vi "Hardware-RegisterFaultPoints.vi"(8 "System State":T3 {"System ADC"."Fan [V]" format="%#_3p"; "System ADC"."Primary B1B2 [V]" format="%#_3p"; "System ADC"."Primary B3B4 [V]" format="%#_3p"; "System ADC"."Primary A3A4 [V]" format="%#_3p"; "System ADC"."Primary A1A2 [V]" format="%#_3p"; "System ADC"."MPRD [V]" format="%#_3p"; "System ADC"."Ext HV B [V]" format="%#_3p"; "System ADC"."Ext HV A [V]" format="%#_3p"; "System ADC"."Pump Zener B [V]" format="%#_3p"; "System ADC"."Pump Zener A [V]" format="%#_3p"; "System ADC"."DI Zener B [V]" format="%#_3p"; "System ADC"."DI Zener A [V]" format="%#_3p"; "System ADC"."Key [V]" format="%#_3p"; "System ADC"."DRVP [V]" format="%#_3p"; "System ADC"."Battery [V]" format="%#_3p"; "System ADC"."FET Driver [V]" format="%#_3p"; "System ADC"."Secondary B1B2 [V]" format="%#_3p"; "System ADC"."Secondary B3B4 [V]" format="%#_3p"; "System ADC"."Secondary A3A4 [V]" format="%#_3p"; "System ADC"."Secondary A1A2 [V]" format="%#_3p"; "System ADC"."Primary Range [V]" format="%#_3p"; "System ADC"."Temp Boost B [C]" format="%#_3p"; "System ADC"."Temp Primary A [C]" format="%#_3p"; "System ADC"."Temp Secondary A [C]" format="%#_3p"; "System ADC"."Temp Fan Intake [C]" format="%#_3p"; "System ADC"."Temp CPU [C]" format="%#_3p"; "System ADC"."Temp DI Zener B [C]" format="%#_3p"; "System ADC"."Temp DI B [C]" format="%#_3p"; "System ADC"."Temp DI Zener A [C]" format="%#_3p"; "System ADC"."Temp DI A [C]" format="%#_3p"; "System ADC"."Temp HH 7-12 [C]" format="%#_3p"; "System ADC"."Temp HH 1-6 [C]" format="%#_3p"; "System ADC"."AI 12 [V]" format="%#_3p"; "System ADC"."AI 11 [V]" format="%#_3p"; "System ADC"."AI 10 [V]" format="%#_3p"; "System ADC"."AI 9 [V]" format="%#_3p"; "System ADC"."AI 8 [V]" format="%#_3p"; "System ADC"."AI 7 [V]" format="%#_3p"; "System ADC"."AI 6 [V]" format="%#_3p"; "System ADC"."AI 5 [V]" format="%#_3p"; "System ADC"."AI 4 [V]" format="%#_3p"; "System ADC"."AI 3 [V]" format="%#_3p"; "System ADC"."AI 2 [V]" format="%#_3p"; "System ADC"."AI 1 [V]" format="%#_3p"}, 9 "DI-B Faults":T1, 10 "DI-A Faults":T1, 11 "HH Status":T6[](array[typedef]) {"On Avg [A]" format="%#_6p"; "Period Avg [A]" format="%#_6p"; "Period Max [A]" format="%#_6p"; "Period Min [A]" format="%#_6p"}) -> ()   [LabVIEW 2016, in "DSI-RT.lvlib"]
uses:
  DSI-RT.lvlib
  <vilib>/Powertrain Controls/Device Drivers/DCM/HH/RT/Status.ctl
  <vilib>/Powertrain Controls/Device Drivers/DCM/Rev0/RT/System State.ctl
  <vilib>/Powertrain Controls/Device Drivers/DCM/Rev0/RT/System ADC.ctl
  <vilib>/Powertrain Controls/Device Drivers/DCM/Rev0/RT/Internal Fault.ctl
  Shared/Typedefs/DI-Faults-Array.ctl
  <vilib>/Powertrain Controls/Device Drivers/DCM/Rev0/FPGA/DI - Faults.ctl
  <vilib>/addons/Software Calibration Management/xSCM/FaultPoint.xnode
  <vilib>/addons/Software Calibration Management/xSCM/CalPoint.xnode
  <vilib>/addons/Software Calibration Management/xSCM/ni_scm.dll
  <vilib>/Powertrain Controls/Device Drivers/DCM/Rev0/RT/DCM - RT.lvclass
  <vilib>/Powertrain Controls/Device Drivers/DCM/HH/RT/DCM - RT - HH.lvlib
  <vilib>/Powertrain Controls/Device Drivers/DCM/Rev0/FPGA/DCM - FPGA.lvlib
  Shared/DSI-Shared.lvlib
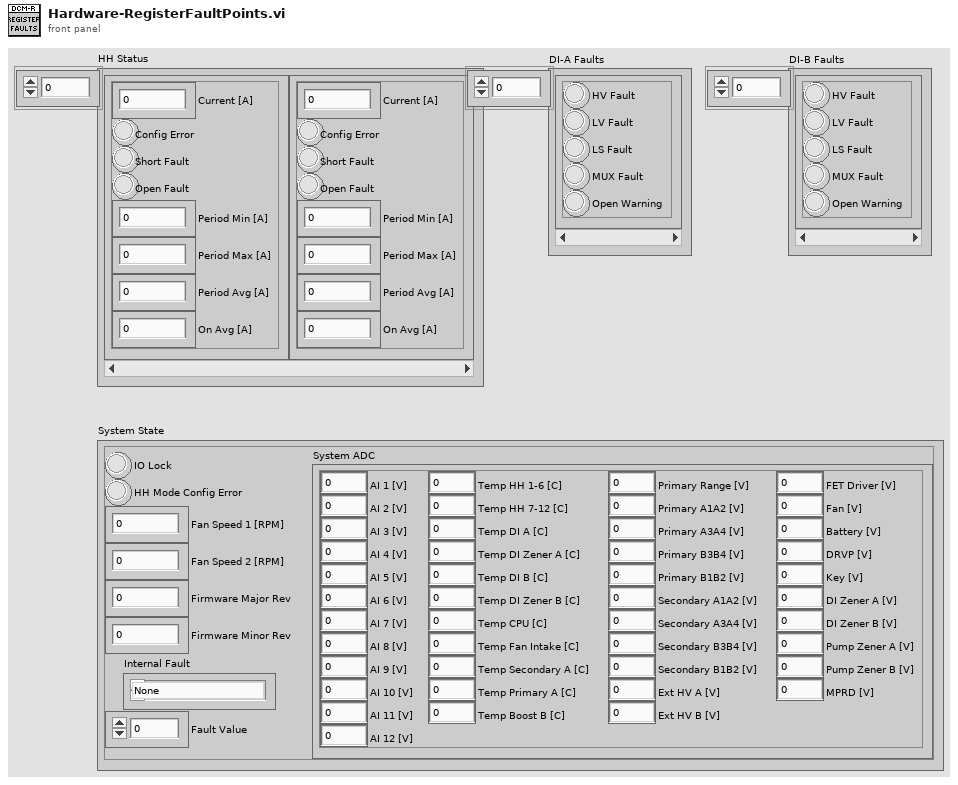
[diagram p1: front panel]
types:
  T1 = typedef "DSI-Shared.lvlib/DI-Faults-Array.ctl" = T2[]
  T2 = typedef "DCM - FPGA.lvlib/DI - Faults.ctl" = cluster{"HV Fault":bool, "LV Fault":bool, "LS Fault":bool, "MUX Fault":bool, "Open Warning":bool}
  T3 = typedef "DCM - RT.lvclass/System State.ctl" = cluster{"System ADC":T4, "IO Lock":bool, "HH Mode Config Error":bool, "Fan Speed 1 [RPM]":sgl, "Fan Speed 2 [RPM]":sgl, "Firmware Major Rev":u16, "Firmware Minor Rev":u16, "Internal Fault":T5, "Fault Value":dbl}
  T4 = typedef "DCM - RT.lvclass/System ADC.ctl" = cluster{"AI 1 [V]":sgl, "AI 2 [V]":sgl, "AI 3 [V]":sgl, "AI 4 [V]":sgl, "AI 5 [V]":sgl, "AI 6 [V]":sgl, "AI 7 [V]":sgl, "AI 8 [V]":sgl, "AI 9 [V]":sgl, "AI 10 [V]":sgl, "AI 11 [V]":sgl, "AI 12 [V]":sgl, "Temp HH 1-6 [C]":sgl, "Temp HH 7-12 [C]":sgl, "Temp DI A [C]":sgl, "Temp DI Zener A [C]":sgl, "Temp DI B [C]":sgl, "Temp DI Zener B [C]":sgl, "Temp CPU [C]":sgl, "Temp Fan Intake [C]":sgl, "Temp Secondary A [C]":sgl, "Temp Primary A [C]":sgl, "Temp Boost B [C]":sgl, "Primary Range [V]":sgl, "Primary A1A2 [V]":sgl, "Primary A3A4 [V]":sgl, "Primary B3B4 [V]":sgl, "Primary B1B2 [V]":sgl, "Secondary A1A2 [V]":sgl, "Secondary A3A4 [V]":sgl, "Secondary B3B4 [V]":sgl, "Secondary B1B2 [V]":sgl, "Ext HV A [V]":sgl, "Ext HV B [V]":sgl, "FET Driver [V]":sgl, "Fan [V]":sgl, "Battery [V]":sgl, "DRVP [V]":sgl, "Key [V]":sgl, "DI Zener A [V]":sgl, "DI Zener B [V]":sgl, "Pump Zener A [V]":sgl, "Pump Zener B [V]":sgl, "MPRD [V]":sgl}
  T5 = typedef "DCM - RT.lvclass/Internal Fault.ctl" = enum32{"None", "Temp HH 1-6", "Temp HH 7-12", "Temp DI A", "Temp DI Zener A", "Temp DI B", "Temp DI Zener B", "Temp Intake", "Temp Primary A", "Temp Secondary A", "Temp Boost B", "Temp CPU", "Low Battery", "Inrush Protection", "A Run Enable", "B Run Enable"}
  T6 = typedef "DCM - RT - HH.lvlib/Status.ctl" = cluster{"Current [A]":sgl, "Config Error":bool, "Short Fault":bool, "Open Fault":bool, "Period Min [A]":sgl, "Period Max [A]":sgl, "Period Avg [A]":sgl, "On Avg [A]":sgl}
  T7 = cluster{"AI 1 [V]":sgl, "AI 2 [V]":sgl, "AI 3 [V]":sgl, "AI 4 [V]":sgl, "AI 5 [V]":sgl, "AI 6 [V]":sgl, "AI 7 [V]":sgl, "AI 8 [V]":sgl, "AI 9 [V]":sgl, "AI 10 [V]":sgl, "AI 11 [V]":sgl, "AI 12 [V]":sgl, "Temp HH 1-6 [C]":sgl, "Temp HH 7-12 [C]":sgl, "Temp DI A [C]":sgl, "Temp DI Zener A [C]":sgl, "Temp DI B [C]":sgl, "Temp DI Zener B [C]":sgl, "Temp CPU [C]":sgl, "Temp Fan Intake [C]":sgl, "Temp Boost A [C]":sgl, "Temp Boost B [C]":sgl, "Temp Boost C [C]":sgl, "Boost Rev [V]":sgl, "Primary A1A2 [V]":sgl, "Primary A3A4 [V]":sgl, "Primary B3B4 [V]":sgl, "Primary B1B2 [V]":sgl, "Secondary A1A2 [V]":sgl, "Secondary A3A4 [V]":sgl, "Secondary B3B4 [V]":sgl, "Secondary B1B2 [V]":sgl, "Ext HV A [V]":sgl, "Ext HV B [V]":sgl, "FET Driver [V]":sgl, "Fan [V]":sgl, "Battery [V]":sgl, "DRVP [V]":sgl, "Key [V]":sgl, "DI Zener A [V]":sgl, "DI Zener B [V]":sgl, "Pump Zener A [V]":sgl, "Pump Zener B [V]":sgl, "MPRD [V]":sgl}
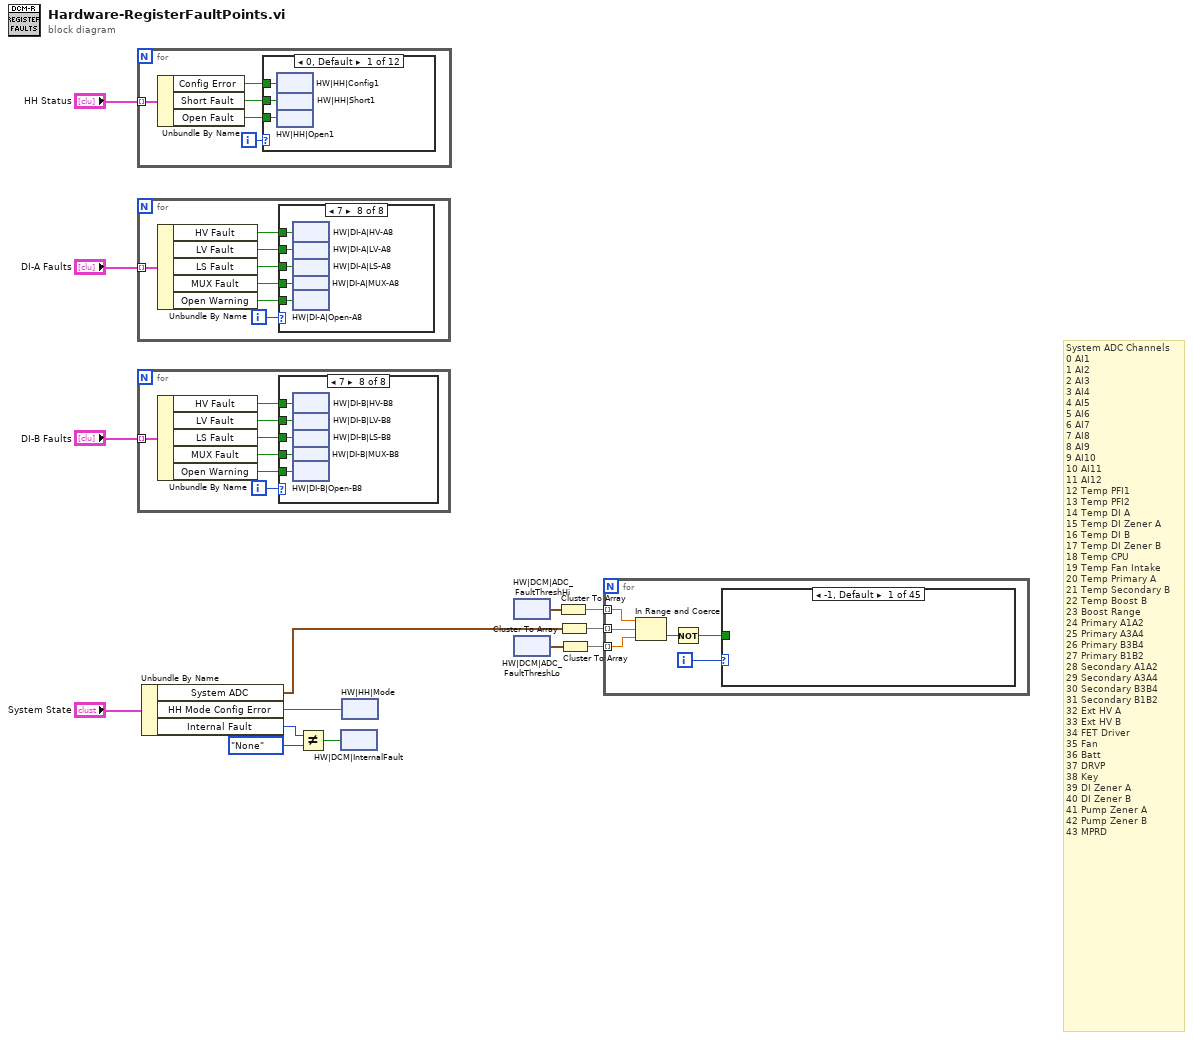
[diagram p0: block diagram]
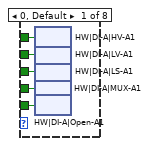
[diagram p2: hidden frame]
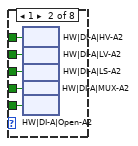
[diagram p3: hidden frame]
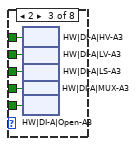
[diagram p4: hidden frame]
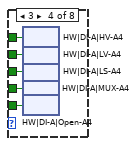
[diagram p5: hidden frame]
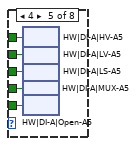
[diagram p6: hidden frame]
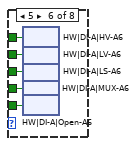
[diagram p7: hidden frame]
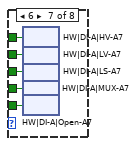
[diagram p8: hidden frame]
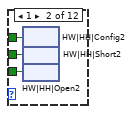
[diagram p9: hidden frame]
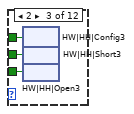
[diagram p10: hidden frame]
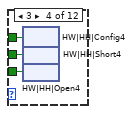
[diagram p11: hidden frame]
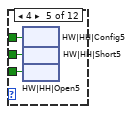
[diagram p12: hidden frame]
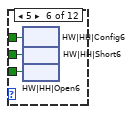
[diagram p13: hidden frame]
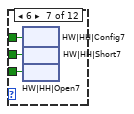
[diagram p14: hidden frame]
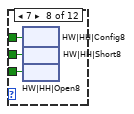
[diagram p15: hidden frame]
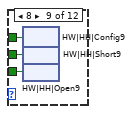
[diagram p16: hidden frame]
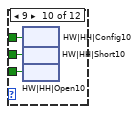
[diagram p17: hidden frame]
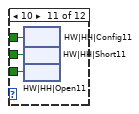
[diagram p18: hidden frame]
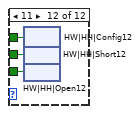
[diagram p19: hidden frame]
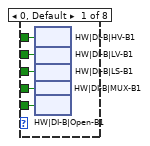
[diagram p20: hidden frame]
diagram:
  # "System ADC Channels\n0\tAI1\n1\tAI2\n2\tAI3\n3\tAI4\n4\tAI5\n5\tAI6\n6\tAI7\n7\tAI8\n8\tAI9\n9\tAI10\n10\tAI11\n11\tAI12\n12\tTemp PFI1\n13\tTemp PFI2\n14\tTemp DI A\n15\tTemp DI Zener A\n16\tTemp DI B\n17\tTemp DI Zener B\n18\tTemp CPU\n19\tTemp Fan Intake\n20\tTemp Primary A\n21\tTemp Secondary B\n22\tTemp Boost B\n23 Boost Range\n24\tPrimary A1A2\n25\tPrimary A3A4\n26\tPrimary B3B4\n27\tPrimary B1B2\n28\tSecondary A1A2\n29\tSecondary A3A4\n30\tSecondary B3B4\n31\tSecondary B1B2\n32\tExt HV A\n33\tExt HV B\n34\tFET Driver\n35 Fan\n36\tBatt\n37\tDRVP\n38\tKey\n39\tDI Zener A\n40\tDI Zener B\n41\tPump Zener A\n42\tPump Zener B\n43\tMPRD"
  n1 = for {
    tunnel: "HH Status" -> [w19] mode=indexing
    i -> [w18]
    n2 = Unbundle By Name(w19) -> ("Config Error"=w17:bool, "Short Fault"=w16:bool, "Open Fault"=w15:bool)
    n3 = case shown="0, Default" w18 {
      tunnel: w17 -> [w22 w37 w52 w67 w82 w97 w112 w127 w142 w157 w172 w187]
      tunnel: w16 -> [w21 w36 w51 w66 w81 w96 w111 w126 w141 w156 w171 w186]
      tunnel: w15 -> [w20 w35 w50 w65 w80 w95 w110 w125 w140 w155 w170 w185]
      frame 0, Default {
        n4 = xnode "HW|HH|Config1"("Fault"=w22) -> ()
        n5 = xnode "HW|HH|Short1"("Fault"=w21) -> ()
        n6 = xnode "HW|HH|Open1"("Fault"=w20) -> ()
      }
      frame 1 {
        n7 = xnode "HW|HH|Config2"("Fault"=w37) -> ()
        n8 = xnode "HW|HH|Short2"("Fault"=w36) -> ()
        n9 = xnode "HW|HH|Open2"("Fault"=w35) -> ()
      }
      frame 2 {
        n10 = xnode "HW|HH|Config3"("Fault"=w52) -> ()
        n11 = xnode "HW|HH|Short3"("Fault"=w51) -> ()
        n12 = xnode "HW|HH|Open3"("Fault"=w50) -> ()
      }
      frame 3 {
        n13 = xnode "HW|HH|Config4"("Fault"=w67) -> ()
        n14 = xnode "HW|HH|Short4"("Fault"=w66) -> ()
        n15 = xnode "HW|HH|Open4"("Fault"=w65) -> ()
      }
      frame 4 {
        n16 = xnode "HW|HH|Config5"("Fault"=w82) -> ()
        n17 = xnode "HW|HH|Short5"("Fault"=w81) -> ()
        n18 = xnode "HW|HH|Open5"("Fault"=w80) -> ()
      }
      frame 5 {
        n19 = xnode "HW|HH|Config6"("Fault"=w97) -> ()
        n20 = xnode "HW|HH|Short6"("Fault"=w96) -> ()
        n21 = xnode "HW|HH|Open6"("Fault"=w95) -> ()
      }
      frame 6 {
        n22 = xnode "HW|HH|Config7"("Fault"=w112) -> ()
        n23 = xnode "HW|HH|Short7"("Fault"=w111) -> ()
        n24 = xnode "HW|HH|Open7"("Fault"=w110) -> ()
      }
      frame 7 {
        n25 = xnode "HW|HH|Config8"("Fault"=w127) -> ()
        n26 = xnode "HW|HH|Short8"("Fault"=w126) -> ()
        n27 = xnode "HW|HH|Open8"("Fault"=w125) -> ()
      }
      frame 8 {
        n28 = xnode "HW|HH|Config9"("Fault"=w142) -> ()
        n29 = xnode "HW|HH|Short9"("Fault"=w141) -> ()
        n30 = xnode "HW|HH|Open9"("Fault"=w140) -> ()
      }
      frame 9 {
        n31 = xnode "HW|HH|Config10"("Fault"=w157) -> ()
        n32 = xnode "HW|HH|Short10"("Fault"=w156) -> ()
        n33 = xnode "HW|HH|Open10"("Fault"=w155) -> ()
      }
      frame 10 {
        n34 = xnode "HW|HH|Config11"("Fault"=w172) -> ()
        n35 = xnode "HW|HH|Short11"("Fault"=w171) -> ()
        n36 = xnode "HW|HH|Open11"("Fault"=w170) -> ()
      }
      frame 11 {
        n37 = xnode "HW|HH|Config12"("Fault"=w187) -> ()
        n38 = xnode "HW|HH|Short12"("Fault"=w186) -> ()
        n39 = xnode "HW|HH|Open12"("Fault"=w185) -> ()
      }
    }
  }
  n40 = for {
    tunnel: "DI-A Faults" -> [w206] mode=indexing
    i -> [w202]
    n41 = Unbundle By Name(w206) -> ("HV Fault"=w205:bool, "LV Fault"=w204:bool, "LS Fault"=w203:bool, "MUX Fault"=w200:bool, "Open Warning"=w201:bool)
    n42 = case shown="7" w202 {
      tunnel: w205 -> [w211 w236 w261 w286 w311 w336 w361 w386]
      tunnel: w204 -> [w210 w235 w260 w285 w310 w335 w360 w385]
      tunnel: w203 -> [w209 w234 w259 w284 w309 w334 w359 w384]
      tunnel: w201 -> [w208 w233 w258 w283 w308 w333 w358 w383]
      tunnel: w200 -> [w207 w232 w257 w282 w307 w332 w357 w382]
      frame 0, Default {
        n43 = xnode "HW|DI-A|HV-A1"("Fault"=w211) -> ()
        n44 = xnode "HW|DI-A|LV-A1"("Fault"=w210) -> ()
        n45 = xnode "HW|DI-A|LS-A1"("Fault"=w209) -> ()
        n46 = xnode "HW|DI-A|MUX-A1"("Fault"=w207) -> ()
        n47 = xnode "HW|DI-A|Open-A1"("Fault"=w208) -> ()
      }
      frame 1 {
        n48 = xnode "HW|DI-A|HV-A2"("Fault"=w236) -> ()
        n49 = xnode "HW|DI-A|LV-A2"("Fault"=w235) -> ()
        n50 = xnode "HW|DI-A|LS-A2"("Fault"=w234) -> ()
        n51 = xnode "HW|DI-A|MUX-A2"("Fault"=w232) -> ()
        n52 = xnode "HW|DI-A|Open-A2"("Fault"=w233) -> ()
      }
      frame 2 {
        n53 = xnode "HW|DI-A|HV-A3"("Fault"=w261) -> ()
        n54 = xnode "HW|DI-A|LV-A3"("Fault"=w260) -> ()
        n55 = xnode "HW|DI-A|LS-A3"("Fault"=w259) -> ()
        n56 = xnode "HW|DI-A|MUX-A3"("Fault"=w257) -> ()
        n57 = xnode "HW|DI-A|Open-A3"("Fault"=w258) -> ()
      }
      frame 3 {
        n58 = xnode "HW|DI-A|HV-A4"("Fault"=w286) -> ()
        n59 = xnode "HW|DI-A|LV-A4"("Fault"=w285) -> ()
        n60 = xnode "HW|DI-A|LS-A4"("Fault"=w284) -> ()
        n61 = xnode "HW|DI-A|MUX-A4"("Fault"=w282) -> ()
        n62 = xnode "HW|DI-A|Open-A4"("Fault"=w283) -> ()
      }
      frame 4 {
        n63 = xnode "HW|DI-A|HV-A5"("Fault"=w311) -> ()
        n64 = xnode "HW|DI-A|LV-A5"("Fault"=w310) -> ()
        n65 = xnode "HW|DI-A|LS-A5"("Fault"=w309) -> ()
        n66 = xnode "HW|DI-A|MUX-A5"("Fault"=w307) -> ()
        n67 = xnode "HW|DI-A|Open-A5"("Fault"=w308) -> ()
      }
      frame 5 {
        n68 = xnode "HW|DI-A|HV-A6"("Fault"=w336) -> ()
        n69 = xnode "HW|DI-A|LV-A6"("Fault"=w335) -> ()
        n70 = xnode "HW|DI-A|LS-A6"("Fault"=w334) -> ()
        n71 = xnode "HW|DI-A|MUX-A6"("Fault"=w332) -> ()
        n72 = xnode "HW|DI-A|Open-A6"("Fault"=w333) -> ()
      }
      frame 6 {
        n73 = xnode "HW|DI-A|HV-A7"("Fault"=w361) -> ()
        n74 = xnode "HW|DI-A|LV-A7"("Fault"=w360) -> ()
        n75 = xnode "HW|DI-A|LS-A7"("Fault"=w359) -> ()
        n76 = xnode "HW|DI-A|MUX-A7"("Fault"=w357) -> ()
        n77 = xnode "HW|DI-A|Open-A7"("Fault"=w358) -> ()
      }
      frame 7 {
        n78 = xnode "HW|DI-A|HV-A8"("Fault"=w386) -> ()
        n79 = xnode "HW|DI-A|LV-A8"("Fault"=w385) -> ()
        n80 = xnode "HW|DI-A|LS-A8"("Fault"=w384) -> ()
        n81 = xnode "HW|DI-A|MUX-A8"("Fault"=w382) -> ()
        n82 = xnode "HW|DI-A|Open-A8"("Fault"=w383) -> ()
      }
    }
  }
  n83 = for {
    tunnel: "DI-B Faults" -> [w413] mode=indexing
    i -> [w409]
    n84 = Unbundle By Name(w413) -> ("HV Fault"=w412:bool, "LV Fault"=w411:bool, "LS Fault"=w410:bool, "MUX Fault"=w407:bool, "Open Warning"=w408:bool)
    n85 = case shown="7" w409 {
      tunnel: w412 -> [w418 w443 w468 w493 w518 w543 w568 w593]
      tunnel: w411 -> [w417 w442 w467 w492 w517 w542 w567 w592]
      tunnel: w410 -> [w416 w441 w466 w491 w516 w541 w566 w591]
      tunnel: w408 -> [w415 w440 w465 w490 w515 w540 w565 w590]
      tunnel: w407 -> [w414 w439 w464 w489 w514 w539 w564 w589]
      frame 0, Default {
        n86 = xnode "HW|DI-B|HV-B1"("Fault"=w418) -> ()
        n87 = xnode "HW|DI-B|LV-B1"("Fault"=w417) -> ()
        n88 = xnode "HW|DI-B|LS-B1"("Fault"=w416) -> ()
        n89 = xnode "HW|DI-B|MUX-B1"("Fault"=w414) -> ()
        n90 = xnode "HW|DI-B|Open-B1"("Fault"=w415) -> ()
      }
      frame 1 {
        n91 = xnode "HW|DI-B|HV-B2"("Fault"=w443) -> ()
        n92 = xnode "HW|DI-B|LV-B2"("Fault"=w442) -> ()
        n93 = xnode "HW|DI-B|LS-B2"("Fault"=w441) -> ()
        n94 = xnode "HW|DI-B|MUX-B2"("Fault"=w439) -> ()
        n95 = xnode "HW|DI-B|Open-B2"("Fault"=w440) -> ()
      }
      frame 2 {
        n96 = xnode "HW|DI-B|HV-B3"("Fault"=w468) -> ()
        n97 = xnode "HW|DI-B|LV-B3"("Fault"=w467) -> ()
        n98 = xnode "HW|DI-B|LS-B3"("Fault"=w466) -> ()
        n99 = xnode "HW|DI-B|MUX-B3"("Fault"=w464) -> ()
        n100 = xnode "HW|DI-B|Open-B3"("Fault"=w465) -> ()
      }
      frame 3 {
        n101 = xnode "HW|DI-B|HV-B4"("Fault"=w493) -> ()
        n102 = xnode "HW|DI-B|LV-B4"("Fault"=w492) -> ()
        n103 = xnode "HW|DI-B|LS-B4"("Fault"=w491) -> ()
        n104 = xnode "HW|DI-B|MUX-B4"("Fault"=w489) -> ()
        n105 = xnode "HW|DI-B|Open-B4"("Fault"=w490) -> ()
      }
      frame 4 {
        n106 = xnode "HW|DI-B|HV-B5"("Fault"=w518) -> ()
        n107 = xnode "HW|DI-B|LV-B5"("Fault"=w517) -> ()
        n108 = xnode "HW|DI-B|LS-B5"("Fault"=w516) -> ()
        n109 = xnode "HW|DI-B|MUX-B5"("Fault"=w514) -> ()
        n110 = xnode "HW|DI-B|Open-B5"("Fault"=w515) -> ()
      }
      frame 5 {
        n111 = xnode "HW|DI-B|HV-B6"("Fault"=w543) -> ()
        n112 = xnode "HW|DI-B|LV-B6"("Fault"=w542) -> ()
        n113 = xnode "HW|DI-B|LS-B6"("Fault"=w541) -> ()
        n114 = xnode "HW|DI-B|MUX-B6"("Fault"=w539) -> ()
        n115 = xnode "HW|DI-B|Open-B6"("Fault"=w540) -> ()
      }
      frame 6 {
        n116 = xnode "HW|DI-B|HV-B7"("Fault"=w568) -> ()
        n117 = xnode "HW|DI-B|LV-B7"("Fault"=w567) -> ()
        n118 = xnode "HW|DI-B|LS-B7"("Fault"=w566) -> ()
        n119 = xnode "HW|DI-B|MUX-B7"("Fault"=w564) -> ()
        n120 = xnode "HW|DI-B|Open-B7"("Fault"=w565) -> ()
      }
      frame 7 {
        n121 = xnode "HW|DI-B|HV-B8"("Fault"=w593) -> ()
        n122 = xnode "HW|DI-B|LV-B8"("Fault"=w592) -> ()
        n123 = xnode "HW|DI-B|LS-B8"("Fault"=w591) -> ()
        n124 = xnode "HW|DI-B|MUX-B8"("Fault"=w589) -> ()
        n125 = xnode "HW|DI-B|Open-B8"("Fault"=w590) -> ()
      }
    }
  }
  n126 = Unbundle By Name("System State") -> ("System ADC"=w1:T4, "HH Mode Config Error"=w11:bool, "Internal Fault"=w4:T5)
  n127 = Not Equal?(x=w4, y=Internal_Fault."None" ("Internal Fault")) -> (x != y?=w2:bool)
  n128 = xnode "HW|DCM|InternalFault"("Fault"=w2) -> ()
  n129 = xnode "HW|HH|Mode"("Fault"=w11) -> ()
  n130 = xnode "HW|DCM|ADC_FaultThreshHi"() -> ("Value"=w8:T7)
  n131 = xnode "HW|DCM|ADC_FaultThreshLo"() -> ("Value"=w9:T7)
  n132 = Cluster To Array(cluster=w8) -> (array=w6:sgl[])
  n133 = Cluster To Array(cluster=w1) -> (array=w7:sgl[])
  n134 = Cluster To Array(cluster=w9) -> (array=w5:sgl[])
  n135 = for {
    tunnel: w7 -> [w617] mode=indexing
    tunnel: w5 -> [w618] mode=indexing
    tunnel: w6 -> [w619] mode=indexing
    i -> [w615]
    n136 = In Range and Coerce(upper limit=w619, x=w617, lower limit=w618) -> (In Range?=w616:bool)  [unwired: 1 out]
    n137 = Not(x=w616) -> (.not. x?=w614:bool)
    n138 = case shown="-1, Default" w615 {
      tunnel: w614 -> [_ w620 w625 w630 w635 w640 w645 w650 w655 w660 w665 w670 w675 w680 w685 w690 w695 w700 w705 w710 w715 w720 w725 w730 w735 w740 w745 w750 w755 w760 w765 w770 w775 w780 w785 w790 w795 w800 w805 w810 w815 w820 w825 w830 w835]
      frame -1, Default {
      }
      frame 0 {
        n139 = xnode "HW|DCM|ADC_AI1"("Fault"=w620) -> ()
      }
      frame 1 {
        n140 = xnode "HW|DCM|ADC_AI2"("Fault"=w625) -> ()
      }
      frame 2 {
        n141 = xnode "HW|DCM|ADC_AI3"("Fault"=w630) -> ()
      }
      frame 3 {
        n142 = xnode "HW|DCM|ADC_AI4"("Fault"=w635) -> ()
      }
      frame 4 {
        n143 = xnode "HW|DCM|ADC_AI5"("Fault"=w640) -> ()
      }
      frame 5 {
        n144 = xnode "HW|DCM|ADC_AI6"("Fault"=w645) -> ()
      }
      frame 6 {
        n145 = xnode "HW|DCM|ADC_AI7"("Fault"=w650) -> ()
      }
      frame 7 {
        n146 = xnode "HW|DCM|ADC_AI8"("Fault"=w655) -> ()
      }
      frame 8 {
        n147 = xnode "HW|DCM|ADC_AI9"("Fault"=w660) -> ()
      }
      frame 9 {
        n148 = xnode "HW|DCM|ADC_AI10"("Fault"=w665) -> ()
      }
      frame 10 {
        n149 = xnode "HW|DCM|ADC_AI11"("Fault"=w670) -> ()
      }
      frame 11 {
        n150 = xnode "HW|DCM|ADC_AI12"("Fault"=w675) -> ()
      }
      frame 12 {
        n151 = xnode "HW|DCM|ADC_Temp-PFI1"("Fault"=w680) -> ()
      }
      frame 13 {
        n152 = xnode "HW|DCM|ADC_Temp-PFI2"("Fault"=w685) -> ()
      }
      frame 14 {
        n153 = xnode "HW|DCM|ADC_Temp-DI-A"("Fault"=w690) -> ()
      }
      frame 15 {
        n154 = xnode "HW|DCM|ADC_Temp-DI-Zener-A"("Fault"=w695) -> ()
      }
      frame 16 {
        n155 = xnode "HW|DCM|ADC_Temp-DI-B"("Fault"=w700) -> ()
      }
      frame 17 {
        n156 = xnode "HW|DCM|ADC_Temp-DI-Zener-B"("Fault"=w705) -> ()
      }
      frame 18 {
        n157 = xnode "HW|DCM|ADC_Temp-CPU"("Fault"=w710) -> ()
      }
      frame 19 {
        n158 = xnode "HW|DCM|ADC_Temp-Fan-Intake"("Fault"=w715) -> ()
      }
      frame 20 {
        n159 = xnode "HW|DCM|ADC_Temp-Primary-A"("Fault"=w720) -> ()
      }
      frame 21 {
        n160 = xnode "HW|DCM|ADC_Temp-Secondary-A"("Fault"=w725) -> ()
      }
      frame 22 {
        n161 = xnode "HW|DCM|ADC_Temp-Boost-B"("Fault"=w730) -> ()
      }
      frame 23 {
        n162 = xnode "HW|DCM|ADC_Boost-Range"("Fault"=w735) -> ()
      }
      frame 24 {
        n163 = xnode "HW|DCM|ADC_Primary-A1A2"("Fault"=w740) -> ()
      }
      frame 25 {
        n164 = xnode "HW|DCM|ADC_Primary-A3A4"("Fault"=w745) -> ()
      }
      frame 26 {
        n165 = xnode "HW|DCM|ADC_Primary-B3B4"("Fault"=w750) -> ()
      }
      frame 27 {
        n166 = xnode "HW|DCM|ADC_Primary-B1B2"("Fault"=w755) -> ()
      }
      frame 28 {
        n167 = xnode "HW|DCM|ADC_Secondary-A1A2"("Fault"=w760) -> ()
      }
      frame 29 {
        n168 = xnode "HW|DCM|ADC_Secondary-A3A4"("Fault"=w765) -> ()
      }
      frame 30 {
        n169 = xnode "HW|DCM|ADC_Secondary-B3B4"("Fault"=w770) -> ()
      }
      frame 31 {
        n170 = xnode "HW|DCM|ADC_Secondary-B1B2"("Fault"=w775) -> ()
      }
      frame 32 {
        n171 = xnode "HW|DCM|ADC_Ext-HV-A"("Fault"=w780) -> ()
      }
      frame 33 {
        n172 = xnode "HW|DCM|ADC_Ext-HV-B"("Fault"=w785) -> ()
      }
      frame 34 {
        n173 = xnode "HW|DCM|ADC_FET-Driver"("Fault"=w790) -> ()
      }
      frame 35 {
        n174 = xnode "HW|DCM|ADC_Fan"("Fault"=w795) -> ()
      }
      frame 36 {
        n175 = xnode "HW|DCM|ADC_Battery"("Fault"=w800) -> ()
      }
      frame 37 {
        n176 = xnode "HW|DCM|ADC_DRVP"("Fault"=w805) -> ()
      }
      frame 38 {
        n177 = xnode "HW|DCM|ADC_Key"("Fault"=w810) -> ()
      }
      frame 39 {
        n178 = xnode "HW|DCM|ADC_DI-Zener-A"("Fault"=w815) -> ()
      }
      frame 40 {
        n179 = xnode "HW|DCM|ADC_DI-Zener-B"("Fault"=w820) -> ()
      }
      frame 41 {
        n180 = xnode "HW|DCM|ADC_Pump-Zener-A"("Fault"=w825) -> ()
      }
      frame 42 {
        n181 = xnode "HW|DCM|ADC_Pump-Zener-B"("Fault"=w830) -> ()
      }
      frame 43 {
        n182 = xnode "HW|DCM|ADC_MPRD"("Fault"=w835) -> ()
      }
    }
  }
